vi "Clip Cross Array.vi"(5 "PathSupreme":T1, 6 "Plate \nDiameter (mm)":dbl, 7 "Cross X dimension\n(cross is square)":dbl, 8 "Origion Array":dbl[][](array[numeric])) -> (3 "PathSupreams":T1[](array[typedef]))   [LabVIEW 2014]
uses:
  Slicer/LVslicer/Slice/TypeDefs/PathSupreme.ctl
  Slicer/LVslicer/Slice/OverhangParam/PSup2SCAN/Sub/VelocityProfile.ctl
  Slicer/LVslicer/Slice/OverhangParam/PSup2SCAN/Sub/PathCut.ctl
  Slicer/LVslicer/Slice/OverhangParam/PSup2SCAN/Sub/Segment.ctl
panel:
  out "min value":dbl
  out "max value":dbl
  out "Array 2":dbl[][](array[numeric])
  out "Origion Output":dbl[][](array[numeric])
  out "#rows":i32
  out "maxY":dbl[][](array[numeric])
  out "indexes":i32[](array[numeric])
  out "Xpoints":dbl[](array[numeric])
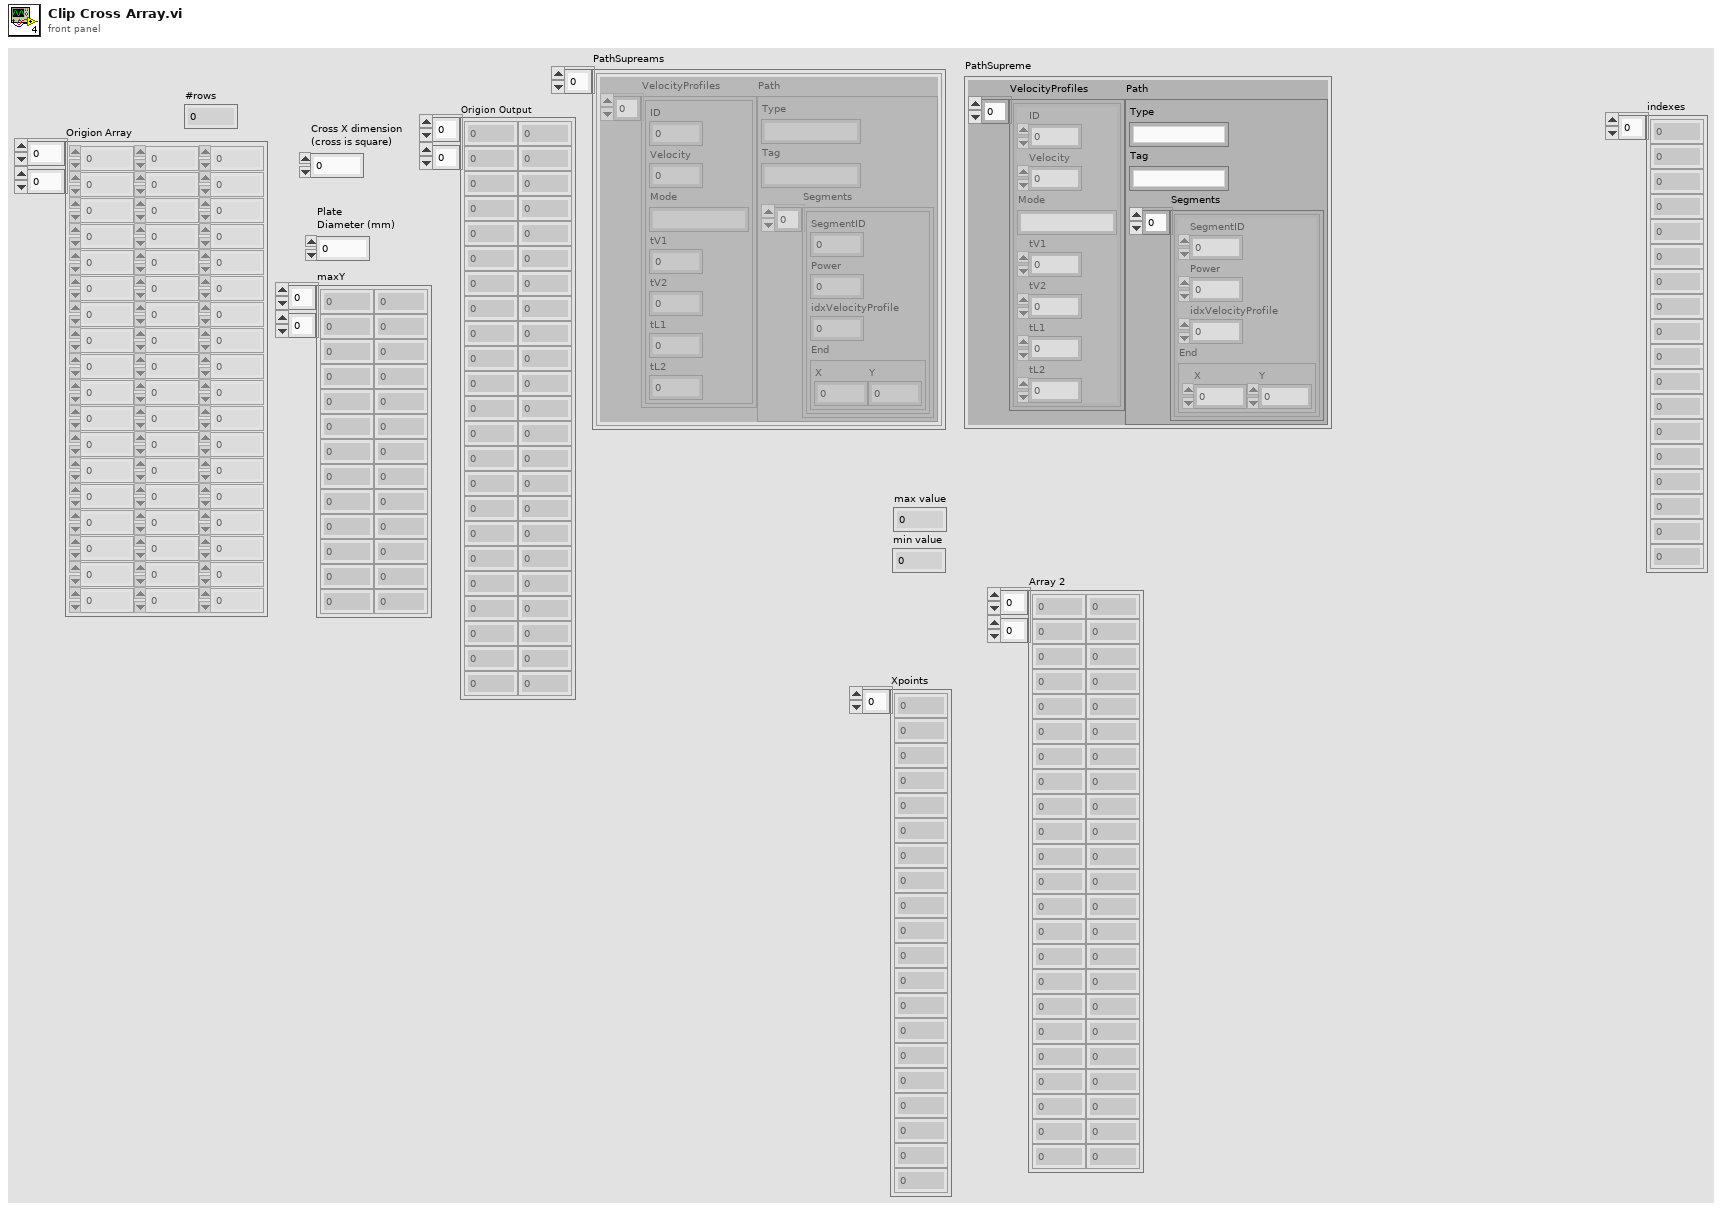
[diagram p1: front panel]
types:
  T1 = typedef "PathSupreme.ctl" = cluster{"VelocityProfiles":T2[], "Path":T3}
  T2 = typedef "VelocityProfile.ctl" = cluster{"ID":u32, "Velocity":dbl, "Mode":string, "tV1":u32, "tV2":u32, "tL1":u32, "tL2":u32}
  T3 = typedef "PathCut.ctl" = cluster{"Type":string, "Tag":string, "Segments":T4[]}
  T4 = typedef "Segment.ctl" = cluster{"SegmentID":u16, "Power":sgl, "idxVelocityProfile":u16, "End":cluster{"X":sgl, "Y":sgl}}
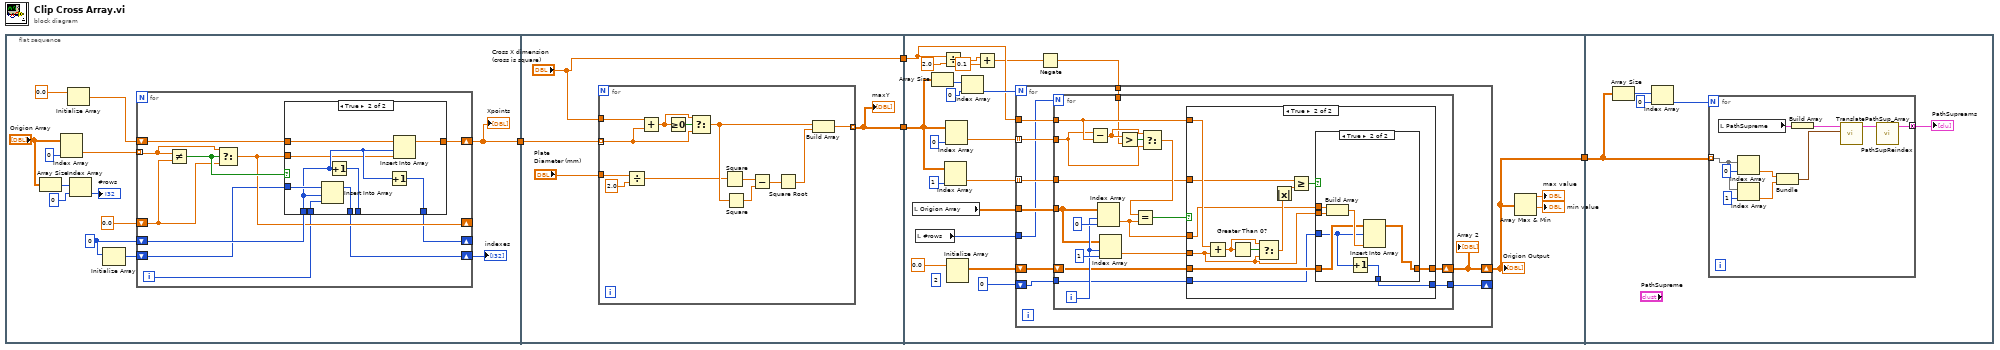
[diagram p0: block diagram]
diagram:
  n1 = flat-sequence {
    tunnel: [w9] -> w4
    tunnel: w4 -> [w43]
    tunnel: [w42] -> w3
    tunnel: ["Cross X dimension\n(cross is square)"] -> w2
    tunnel: w3 -> [w73]
    tunnel: w2 -> [w65]
    tunnel: [w60] -> w1
    tunnel: w1 -> [w132]
    frame #0 {
      w14 = 0
      n2 = Array Size(array="Origion Array") -> (size(s)=w8:i32[])
      n3 = Index Array(array="Origion Array", index (col)=0 ("disabled index (col)")) -> (element=w11:dbl[])  [unwired: 1 in]
      n4 = Initialize Array(0.0) -> (w15:dbl[])  [unwired: 1 in]
      n5 = Index Array(array=w8, index=0 ("disabled index (col)")) -> (element=→"#rows":i32)
      n6 = Initialize Array(w14) -> (w13:i32[])  [unwired: 1 in]
      n7 = for {
        tunnel: w11 -> [w28] mode=indexing
        shift-right: [w24] -> _
        shift-left: 0.0 -> [w26]
        shift-right: [w18] -> _
        shift-left: w14 -> [w25]
        shift-right: [w19] -> w9
        shift-left: w15 -> [w20]
        shift-right: [w21] -> w12
        shift-left: w13 -> [w23]
        i -> [w22]
        n8 = Not Equal?(x=w28, y=w26) -> (x != y?=w27:bool)
        n9 = Select(t=w28, s=w27, f=w26) -> (s? t:f=w24:dbl)
        n10 = case shown="True" w27 {
          tunnel: w25 -> [w29 w34]
          tunnel: [w29 w35] -> _
          tunnel: w24 -> [_ w32]
          tunnel: [w30 w36] -> w19
          tunnel: w23 -> [w31 w40]
          tunnel: w22 -> [_ w39]
          tunnel: [w31 w38] -> w21
          tunnel: w20 -> [w30 w37]
          tunnel: [w29 w33] -> w18
          frame False {
          }
          frame True {
            n11 = Insert Into Array(array=w40, index=w34, new element=w39) -> (w38:i32[])
            n12 = Increment(x=w34) -> (x+1=w35:i32)
            n13 = Increment(x=w34) -> (x+1=w33:i32)
            n14 = Insert Into Array(array=w37, index=w34, new element=w32) -> (w36:dbl[])
          }
        }
      }
      "indexes" <- w12
      "Xpoints" <- w9
    }
    frame #1 {
      n15 = for {
        tunnel: w43 -> [w55] mode=indexing
        tunnel: "Plate \nDiameter (mm)" -> [w50]
        tunnel: [w54] -> w42 mode=indexing
        tunnel: "Cross X dimension\n(cross is square)" -> [w48]
        n16 = Divide(x=w50, y=2.0) -> (x/y=w46:dbl)
        n17 = Add(x=w48, y=w55) -> (x+y=w56:dbl)
        n18 = Greater Or Equal To 0?(x=w56) -> (x >= 0?=w57:bool)
        n19 = Select(t=w56, s=w57, f=w55) -> (s? t:f=w47:dbl)
        n20 = Square(x=w46) -> (x^2=w52:dbl)
        n21 = Square(x=w47) -> (x^2=w51:dbl)
        n22 = Subtract(x=w52, y=w51) -> (x-y=w53:dbl)
        n23 = Square Root(x=w53) -> (sqrt(x)=w49:dbl)
        n24 = Build Array(w47, w49) -> (w54:dbl[])
      }
      "maxY" <- w42
    }
    frame #2 {
      (unwired) 2 ("dimension size")
      n25 = local read "Origion Array"() -> (w71:dbl[][])
      n26 = local read "#rows"() -> (w68:i32)
      n27 = Array Size(array=w73) -> (size(s)=w79:i32[])
      n28 = Divide(x=w65, y=2.0) -> (x/y=w64:dbl)
      n29 = Index Array(array=w73, index (col)=1 ("disabled index (col)")) -> (element=w72:dbl[])  [unwired: 1 in]
      n30 = Index Array(array=w73, index (col)=0 ("disabled index (col)")) -> (element=w75:dbl[])  [unwired: 1 in]
      n31 = Initialize Array(0.0) -> (w70:dbl[][])  [unwired: 2 in]
      n32 = Index Array(array=w79, index=0 ("disabled index (col)")) -> (element=w77:i32)
      n33 = Add(x=w64, y=0.1) -> (x+y=w62:dbl)
      n34 = Negate(x=w62) -> (-x=w61:dbl)
      n35 = for {
        N: w77 -> [_]
        tunnel: w71 -> [w89]
        tunnel: w75 -> [w88] mode=indexing
        shift-right: [w86] -> w60
        shift-left: w70 -> [w87]
        tunnel: w72 -> [w85] mode=indexing
        tunnel: w65 -> [w84]
        tunnel: w68 -> [w83]
        shift-right: [w81] -> _
        shift-left: 0 -> [w82]
        tunnel: w61 -> [w80]
        n36 = for {
          N: w83 -> [_]
          tunnel: w89 -> [w100]
          tunnel: w88 -> [w91]
          shift-right: [w97] -> w86
          shift-left: w87 -> [w98]
          tunnel: w85 -> [w96]
          tunnel: w84 -> [w92]
          tunnel: w82 -> [w94]
          tunnel: [w93] -> w81
          tunnel: w80 -> [w90]
          i -> [w101]
          n37 = Subtract(x=w91, y=w92) -> (x-y=w105:dbl)
          n38 = Index Array(array=w100, index (row)=w101, index (col)=0 ("disabled index (col)")) -> (element=w95:dbl)
          n39 = Index Array(array=w100, index (row)=w101, index (col)=1 ("disabled index (col)")) -> (element=w99:dbl)
          n40 = Greater?(x=w105, y=w90) -> (0:w106:bool)
          n41 = Select(t=w105, s=w106, f=w91) -> (s? t:f=w104:dbl)
          n42 = Equal?(x=w104, y=w95) -> (x = y?=w103:bool)
          n43 = case shown="True" w103 {
            tunnel: w99 -> [_ w113]
            tunnel: w98 -> [w109 w115]
            tunnel: [w109 w116] -> w97
            tunnel: w96 -> [_ w120]
            tunnel: w92 -> [_ w122]
            tunnel: w95 -> [_ w112]
            tunnel: w94 -> [w108 w114]
            tunnel: [w108 w111] -> w93
            frame False {
            }
            frame True {
              n44 = Add(x=w122, y=w113) -> (x+y=w119:dbl)
              n45 = Greater Than 0?(x=w119) -> (x > 0?=w121:bool)
              n46 = Select(t=w119, s=w121, f=w113) -> (s? t:f=w118:dbl)
              n47 = Absolute Value(x=w118) -> (abs(x)=w110:dbl)
              n48 = Greater Or Equal?(x=w120, y=w110) -> (x >= y?=w117:bool)
              n49 = case shown="True" w117 {
                tunnel: [w124 w127] -> w116
                tunnel: w115 -> [w124 w128]
                tunnel: w114 -> [w123 w126]
                tunnel: w113 -> [_ w131]
                tunnel: w112 -> [_ w130]
                tunnel: [w123 w125] -> w111
                frame False {
                }
                frame True {
                  n50 = Build Array(w130, w131) -> (w129:dbl[])
                  n51 = Increment(x=w126) -> (x+1=w125:i32)
                  n52 = Insert Into Array(array=w128, index (row)=w126, new element=w129) -> (w127:dbl[][])  [unwired: 1 in]
                }
              }
            }
          }
        }
        "Array 2" <- w86
      }
      "Origion Output" <- w60
      n53 = Array Max & Min(array=w60) -> (max value=→"max value":dbl, min value=→"min value":dbl)  [unwired: 2 out]
    }
    frame #3 {
      n54 = Array Size(array=w132) -> (size(s)=w133:i32[])
      n55 = Index Array(array=w133, index=0) -> (element=w135:i32)
      n56 = for {
        N: w135 -> [_]
        tunnel: w132 -> [w146] mode=indexing
        tunnel: [w138] -> w136 mode=concatenating
        n57 = local read "PathSupreme"() -> (w140:T1)
        n58 = Index Array(array=w146, index=0) -> (element=w142:dbl)
        n59 = Index Array(array=w146, index=1) -> (element=w143:dbl)
        n60 = Bundle(w142, w143) -> (w141:cluster{dbl, dbl})  [unwired: 1 in]
        n61 = Build Array(w140) -> (w139:T1[])
        n62 = call "TranslatePathSup_Array.vi"("Offset"=w141, "PathSupsIn"=w139) -> ("PathSupsOut"=w137:T1[])  [unwired: 9 in]
        n63 = call "PathSupReindex.vi"("PathSupremes"=w137) -> ("PathSupOut"=w138:T1[])  [unwired: 10 in]
      }
      "PathSupreams" <- w136
    }
  }
